vi "New-Main.vi"() -> ()   [LabVIEW 2019]
uses:
  <vilib>/userdefined/High Color/IMAQdx.ctl
  <vilib>/Platform/TimedLoop/XDataNode/nitl_modes.ctl
  <vilib>/Platform/TimedLoop/XDataNode/timing_clust.ctl
  <vilib>/Platform/TimedLoop/XDataNode/wakeup.ctl
  <vilib>/UPVI/lvhdf5/dataset.llb/LVH5D Operation.ctl
  <vilib>/Utility/miscctls.llb/LVRectTypeDef.ctl
  <vilib>/UPVI/lvhdf5/attribute.llb/LVH5A Operation.ctl
  <vilib>/UPVI/lvhdf5/group.llb/H5G_obj_t.ctl
  <vilib>/MakerHub/LINX/Public/Peripherals/Digital/Digital Read 1 Chan.vi
  03419f7f-1d90-4d41-b19f-f0295c63df66.vi
  <vilib>/MakerHub/LINX/Public/Peripherals/PWM/PWM Set Duty Cycle 1 Chan.vi
  <vilib>/UPVI/lvhdf5/identifier.llb/Not an HDF5 Refnum Constant.vi
  <vilib>/MakerHub/LINX/Public/Peripherals/Digital/Digital Read N Chans.vi
  <vilib>/UPVI/lvhdf5/common.llb/To HDF5 Ref.vi
  <vilib>/MakerHub/LINX/Private/Local IO/LinxDigitalRead.vi
  <vilib>/MakerHub/LINX/Public/Utilities/Check Channel.vi
  <vilib>/MakerHub/LINX/Public/Utilities/Open Serial.vi
  <vilib>/MakerHub/LINX/Private/Utilties/Generate Error.vi
  <vilib>/Utility/file.llb/Read Delimited Spreadsheet (DBL).vi
  <vilib>/MakerHub/LINX/Public/Peripherals/PWM/PWM Set Duty Cycle N Chans.vi
  <vilib>/UPVI/lvhdf5/group.llb/OpenCreateGroup (String).vi
  <vilib>/Utility/VariantDataType/GetClusterInfo.vi
  <vilib>/Utility/VariantDataType/GetTypeInfo.vi
  <vilib>/UPVI/lvhdf5/utility.llb/Select HDF5 Dialog.vi
  <vilib>/UPVI/lvhdf5/utility.llb/Select HDF5 Dialog (Object Only).vi
  <vilib>/UPVI/lvhdf5/dataset.llb/Simple H5Dwrite (Variant).vi
  <vilib>/UPVI/lvhdf5/attribute.llb/Write Multiple Attributes.vi
  <vilib>/UPVI/lvhdf5/dataset.llb/H5Dclose.vi
  <vilib>/platform/TimedLoop/XDataNode/XDataNode.xnode
  <vilib>/UPVI/lvhdf5/dataset.llb/Write Dataset with Attributes.xnode
  <vilib>/UPVI/lvhdf5/library.llb/HDF5 Ref.ctl
  <vilib>/UPVI/lvhdf5/attribute.llb/Cluster to Attribute Array.xnode
  <vilib>/UPVI/lvhdf5/dataset.llb/Simple H5Dwrite.xnode
  <vilib>/Platform/TimedLoop/XDataNode/XDNodeRunTimeDep.lvlib
  <vilib>/vision/driver/NI_Vision_Acquisition_Software.lvlib
  <vilib>/MakerHub/LINX/LMH-LINX.lvlib
  <vilib>/Utility/error.llb/Error Cluster From Error Code.vi
  <vilib>/UPVI/lvhdf5/dataset.llb/OpenCreateReplace Dataset by Element Type.vi
  <vilib>/UPVI/lvhdf5/dataspace.llb/H5Sselect_hyperslab.vi
  <vilib>/UPVI/lvhdf5/dataset.llb/H5Dwrite (Variant).vi
  <vilib>/UPVI/lvhdf5/dataset.llb/H5Dget_space.vi
  <vilib>/UPVI/lvhdf5/attribute.llb/private/LVH5AwriteWDTAttrs.vi
  <vilib>/UPVI/lvhdf5/dataspace.llb/H5Sclose.vi
  <vilib>/UPVI/lvhdf5/file.llb/LVH5F Operation.ctl
  <vilib>/UPVI/lvhdf5/utility.llb/Select HDF5 Dialog (File and Object).vi
  <vilib>/Utility/VariantDataType/VariantType.lvlib
panel:
  out "output":dbl[](array[numeric])
  out "motor fb":dbl
  in  "stop":bool
  in  "attributes cluster":T1
  out "CW/CCW":bool
  out "x-y":u32
  out "Trial #":i32[](array[numeric])
  out "stimulus":bool
  out "Timers":dbl[](array[numeric])
  out "% In Exit":dbl[](array[numeric])
  in  "Controls":T2={"Start"=FALSE, "Stop"=FALSE, "success"=FALSE, "set"=FALSE, "fail"=FALSE, "Save Data"=FALSE, "poop count"=0, "Rodent ID"=1, "Correct color"=enum."UV"}
  in  "Settings":T3(tab)
  in  "trial settings":T4={"Num Trials"=6, "Trial Duration (s)"=90, "ITI (s)"=20, "incorrect ITI (s)"=5, "Total Timeout (s)"=900} {"incorrect ITI (s)" min=1 step=1; "Total Timeout (s)" min=1 step=1; "ITI (s)" min=1 step=1; "Num Trials" min=2 step=2; "Trial Duration (s)" min=1 step=1}
  in  "dir":T5={"Data Output Directory"=path "D:/pdroft", "Session Name"="default"}
  in  "habituation":bool
  in  "feedback":T6={"motor feedback mode"=enum."constant", "min motor feedback"=0.1, "max motor feedback"=0.5, "max led feedback"=1.0, "colormap"=path "C:/Program Files/PDROFT/data/colormap_test121219e.txt"} {"min motor feedback" min=0.0 max=1.0; "max led feedback" min=0.0 max=1.0; "max motor feedback" min=0.0 max=1.0}
  in  "ROI":T7
  in  "vid bandpass":T8={"low1"=1, "high1"=7, "low2"=27, "high2"=100}
  in  "I/O":T10={"Vid In"="cam0", "record raw video?"=FALSE, "record filtered video?"=FALSE, "microcontroller Serial Port"="COM4", "Disable physical start butn"=FALSE}
  in  "exits":T11={"hab scale"=0.7, "exit radius (cm)"=12.5, "% required in exit"=42.0}
  in  "save settings to ini at close":bool
  in  "load settings from ini at start":bool
  out "Image":T12(plugin-control)
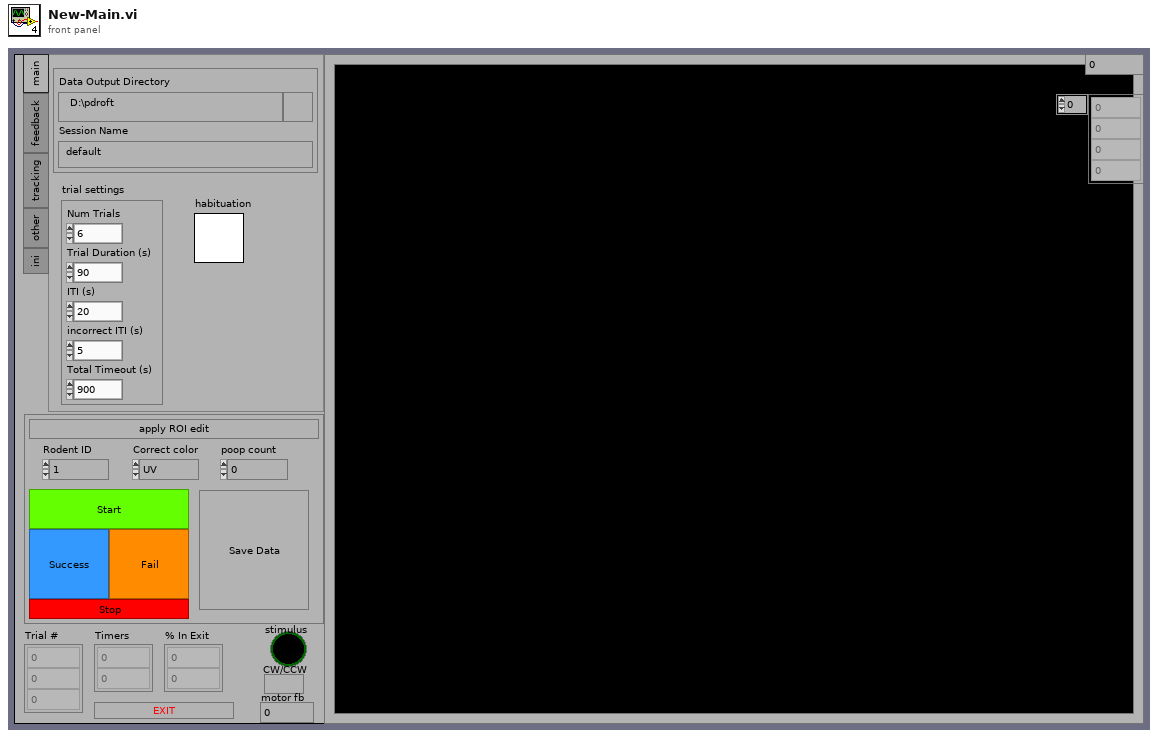
[diagram p1: front panel]
types:
  T1 = cluster{"timestamp":string, "ID":string, "correct color":string, "poop count":string, "trial settings":string, "motor settings":string, "max led fb":string, "colormap":string, "vid bandpass":string, "exit settings":string, "platform":string, "px2cm":string}
  T2 = cluster{"Start":bool, "Stop":bool, "success":bool, "set":bool, "fail":bool, "Save Data":bool, "poop count":i8, "Rodent ID":i32, "Correct color":enum16{"UV", "Green"}}
  T3 = enum32{"main", "feedback", "tracking", "other", "ini"}
  T4 = cluster{"Num Trials":i32, "Trial Duration (s)":i32, "ITI (s)":i32, "incorrect ITI (s)":i32, "Total Timeout (s)":i32}
  T5 = cluster{"Data Output Directory":path, "Session Name":string}
  T6 = cluster{"motor feedback mode":enum16{"constant", "time still"}, "min motor feedback":dbl, "max motor feedback":dbl, "max led feedback":dbl, "colormap":path}
  T7 = cluster{"Global Rectangle":i32[], "Contours":cluster{"Contour Type":u32, "ROI Type":u32, "Points":i32[]}[]}
  T8 = cluster{"low1":i32, "high1":i32, "low2":i32, "high2":i32}
  T9 = typedef "IMAQdx.ctl" = refnum<k21>
  T10 = cluster{"Vid In":T9, "record raw video?":bool, "record filtered video?":bool, "microcontroller Serial Port":refnum<visa-resource-name>, "Disable physical start butn":bool}
  T11 = cluster{"hab scale":dbl, "exit radius (cm)":dbl, "% required in exit":dbl}
  T12 = typedef "IMAQ Image.ctl" = refnum<image>
  T13 = typedef "XDNodeRunTimeDep.lvlib/nitl_modes.ctl" = enum32{"No Change", "Process missed periods, maintain original phase", "Discard missed periods, maintain original phase", "Process missed periods, ignore original phase", "Discard missed periods, ignore original phase"}
  T14 = enum8{"Enabled", "Disabled", "Disabled and Grayed Out"}
  T15 = typedef "LVRectTypeDef.ctl" = cluster{"Left":i16, "Top":i16, "Right":i16, "Bottom":i16}
  T16 = cluster{"Behavior":enum32{"Invalid", "Default", "Floating", "Floating/Auto-Hide", "Modal"}, "Position":T15, "Center":bool, "Title":string}
  T17 = typedef "LVH5F Operation.ctl" = enum16{"open", "open or create", "create or replace", "create or replace (with confirmation)", "create", "open (read only)"}
  T18 = typedef "LVH5D Operation.ctl" = enum16{"open", "replace", "create", "open or create", "create or replace", "create or replace with confirmation"}
  T19 = typedef "H5G_obj_t.ctl" = i32
  T20 = cluster{"Object Types (any)":T19[], "Object Pattern":string}
  T21 = typedef "LVH5A Operation.ctl" = enum16{"open", "replace", "create", "open or create", "create or replace", "create or replace with confirmation"}
  T22 = cluster{"Session Timer":dbl, "Trial Timer":dbl, "Trial #":dbl, "Correction #":dbl, "Omission":dbl, "CentroidX":dbl, "CentroidY":dbl, "%Correct":dbl, "%Incorrect":dbl, "R":dbl, "G":dbl, "B":dbl, "W":dbl, "M":dbl, "Total":dbl}
  T23 = typedef "XDNodeRunTimeDep.lvlib/timing_clust.ctl" = cluster{"Expected End [f-1]":u64, "Actual End [f-1]":u64, "Finished Late? [f-1]":bool, "Expected End [i-1]":u64, "Actual End [i-1]":u64, "Finished Late? [i-1]":bool, "Expected Start [i]":u64, "Actual Start [i]":u64, "Expected Start [f]":u64, "Actual Start [f]":u64, "Source Name":string, "Structure Name":string, "Period":i64, "Deadline":i64, "Offset":i64, "Start":i64, "Priority":i32, "Timeout":i32, "Mode":T13, "Wakeup Reason":T24, "Error":errorcluster, "Source Type":string, "Secondary Source Type":string, "Global End Time":u64, "Global Start Time":u64, "Frame Duration":u64, "Iteration Duration":u64, "Assigned CPU":i32, "I/O Scan Engine Mode":u32}
  T24 = typedef "XDNodeRunTimeDep.lvlib/wakeup.ctl" = enum32{"Normal", "Aborted", "Asynchronous wakeup", "Timing source error", "Timed loop error", "Timeout"}
  T25 = enum32{"invalid app kind", "Development System", "Run Time System", "Student Edition", "Embedded LabVIEW", "Evaluation", "Custom"}
  T26 = typedef "Image Type" = u32
  T27 = typedef "LMH-LINX.lvlib/LINX Ref.ctl" = cluster{"IO":T28, "Interface":T29, "LINX Device Config":T30}
  T28 = typedef "LMH-LINX.lvlib/Platform.ctl" = enum16{"Remote", "Local"}
  T29 = typedef "LMH-LINX.lvlib/Interface.ctl" = enum16{"Serial", "TCP"}
  T30 = typedef "LMH-LINX.lvlib/Device.lvlib/LINX Device Config.ctl" = cluster{"Interface":T29, "COM Port":refnum<visa-resource-name>, "TCP Configuration":T31, "Device Family":u8, "Device ID":u8, "Device Name":string, "TCP Ref":refnum<k5>, "Channels":T32}
  T31 = typedef "LMH-LINX.lvlib/Device.lvlib/TCP Config.ctl" = cluster{"IP Address":string, "Port":u16}
  T32 = typedef "LMH-LINX.lvlib/Channels.ctl" = cluster{"DI":u8[], "DO":u8[], "AI":u8[], "AO":u8[], "PWM":u8[], "QE":u8[], "UART":u8[], "I2C 2":u8[], "SPI":u8[], "CAN":u8[], "Servo":u8[], "AI Ref (V)":dbl, "AI Resolution (Bits)":u8, "AO Ref (V)":dbl, "AO Resolution (Bits)":u8}
  T33 = cluster{"Trial#":dbl, "Correction#":dbl, "Omission":dbl, "CorrectX":dbl, "CorrectY":dbl, "IncorrectX":dbl, "IncorrectY":dbl, "CW/CCW":dbl}
  T34 = typedef "IMAQ AVI2 Refnum.ctl" = refnum<k20>
  T35 = cluster{"Trial#":dbl, "Correction#":dbl, "Omission":dbl, "CorrectX":dbl, "CorrectY":dbl, "IncorrectX":dbl, "IncorrectY":dbl, "CW/CCW":dbl}[]
  T36 = cluster{"center":dbl[], "center":dbl[], "hab rad":dbl, "Timers":dbl[]}
  T37 = cluster{"px2cm":dbl, "center":dbl[], "rad":dbl, "hab rad":dbl, "exit rad":dbl}
  T38 = cluster{"correct exit":dbl[], "incorrect exit":dbl[], "exit rad":dbl, "exit angles":dbl[]}
  T39 = typedef "HDF5 Ref.ctl" = refnum<k1>
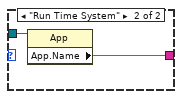
[diagram p3: hidden frame]
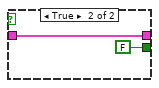
[diagram p4: hidden frame]
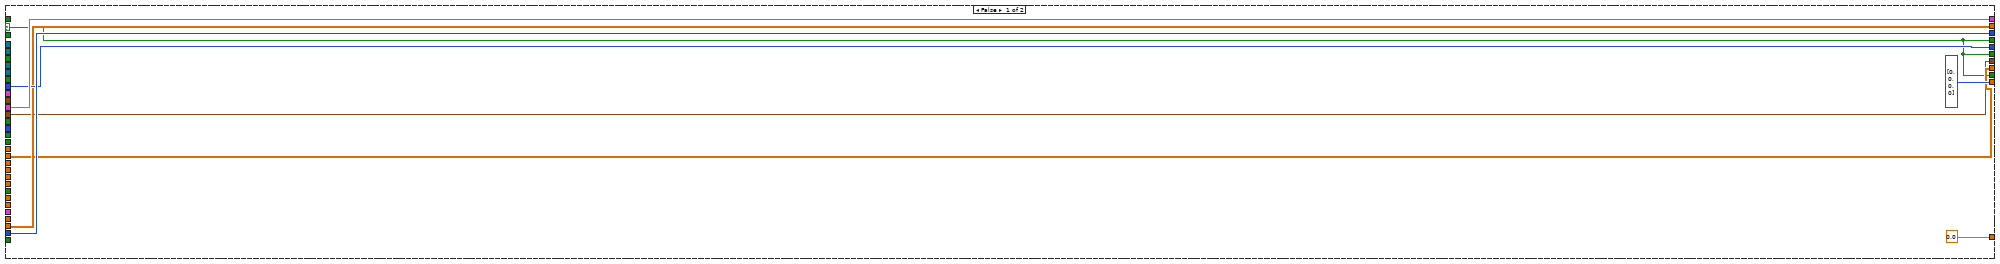
[diagram p9: hidden frame]
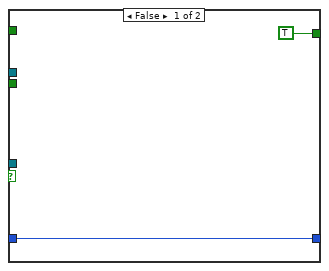
[diagram p11: hidden frame]
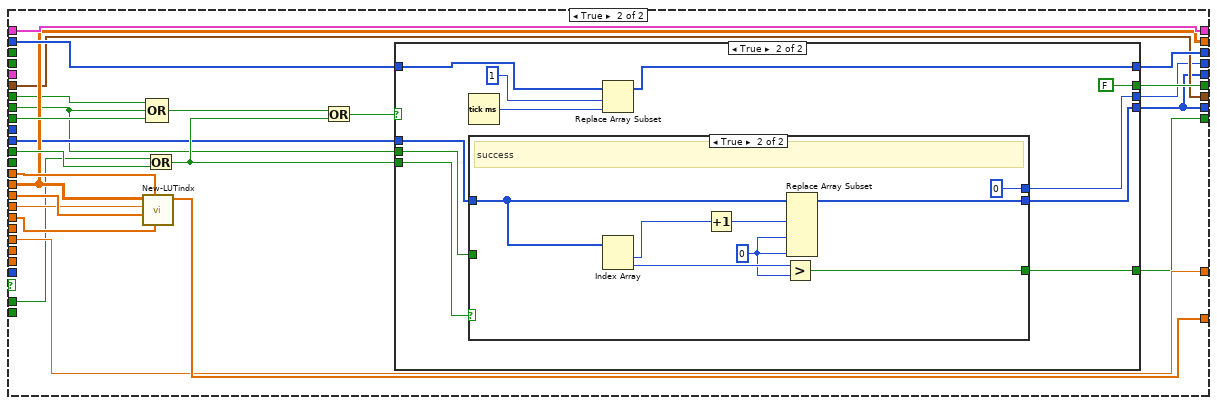
[diagram p16: hidden frame]
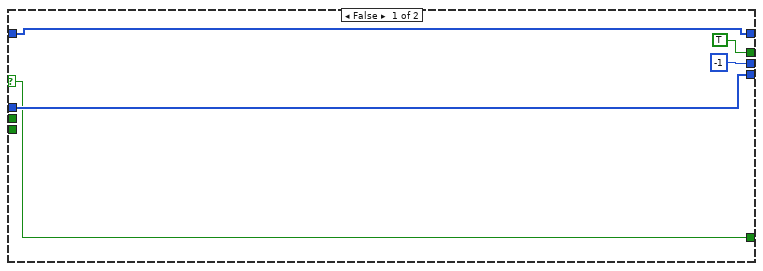
[diagram p17: hidden frame]
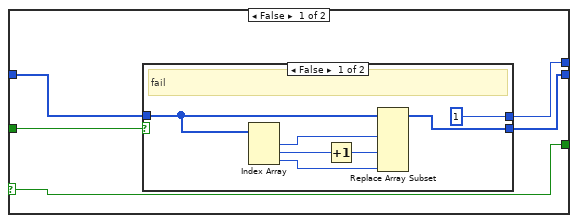
[diagram p18: hidden frame]
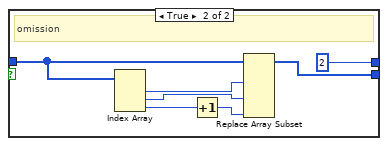
[diagram p19: hidden frame]
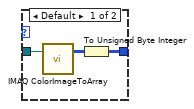
[diagram p20: hidden frame]
diagram:
  n1 = flat-sequence {
    tunnel: [w5] -> w2
    tunnel: [w4] -> w1
    tunnel: w2 -> [w1170]
    tunnel: w1 -> [w1169]
    frame #0 {
      n2 = property class="App"() -> (reference out=w8:refnum<vi>, "App.Kind"=w9:T25)  [unwired: 2 in, 1 out]
      n3 = case shown="\"Development System\", Default" w9 {
        tunnel: w8 -> [_ w16]
        tunnel: [w14 w15] -> w6
        frame "Development System", Default {
          n4 = property class="VI"() -> ("Name"=w14:string)  [unwired: 2 in, 2 out]
        }
        frame "Run Time System" {
          n5 = property class="App"(reference=w16) -> ("App.Name"=w15:string)  [unwired: 1 in, 2 out]
        }
      }
      n6 = control-ref of="Settings"() -> (w7:refnum<vi>)
      n7 = property class="TabCtl (strict)"(reference=w7) -> ("Pages"=w4:refnum<vi>[])  [unwired: 1 in, 2 out]
      n8 = call "Generate INI file path.vi"("VI or App Name"=w6) -> ("appended path"=w5:path)
      n9 = case shown="True" "load settings from ini at start" {
        tunnel: w5 -> [_ w11]
        tunnel: w4 -> [_ w10]
        frame False {
        }
        frame True {
          n10 = for {
            tunnel: w11 -> [w13]
            tunnel: w10 -> [w12] mode=indexing
            n11 = call "my Read Controls on Tab from Config File.vi"("Page Refnum"=w12, "configuration file path"=w13) -> ()  [unwired: 4 in, 2 out]
          }
        }
      }
    }
    frame #1 {
      n12 = control-ref of="Image"() -> (w18:refnum<vi>)
      n13 = property class="ImageControl"(reference=w18, "ROI"="ROI") -> ()  [unwired: 1 in, 2 out]
    }
    frame #2 {
      w33 = dbl[] [0.0, 0.0] ("Timers")
      w27 = FALSE
      w36 = T26 0 items=["Grayscale (U8)", "Grayscale (I16)", "Grayscale (SGL)", "Complex (CSG)", "RGB (U32)", "HSL (U32)", "RGB (U64)", "Grayscale (U16)"] ("Image Type")
      n14 = property on="Timers" class="Arr (strict)"("Value"=w33) -> ()  [unwired: 2 in, 2 out]
      n15 = property on="% In Exit" class="Arr (strict)"("Value"=w33) -> ()  [unwired: 2 in, 2 out]
      n16 = Unbundle("I/O") -> ("Vid In"=w47:T9, "record raw video?"=w38:bool, "record filtered video?"=w22:bool, "microcontroller Serial Port"=w23:refnum<visa-resource-name>, "Disable physical start butn"=w19:bool)
      n17 = call-poly <vilib>:"Open.vi"("Serial Port"=w23) -> ("Error Out"=w26:errorcluster, "LINX Resource"=w29:T27)  [unwired: 8 in, 1 out]
      n18 = call <vilib>:"IMAQdx Open Camera.vi"("Session In"=w47) -> ("Session Out"=w48:T9)  [unwired: 9 in, 1 out]
      n19 = call <vilib>:"IMAQdx Configure Grab.vi"("Session In"=w48) -> ("Session Out"=w43:T9)  [unwired: 9 in, 1 out]
      n20 = call <vilib>:"General Error Handler.vi"("[error source] (\" \")"="microcontroller connection" ("[error source] (\" \")"), "error in (no error)"=w26) -> ("error?"=w25:bool)  [unwired: 9 in, 4 out]
      n21 = call "IMAQ Create"("Image Name"="untitled0", "Image Type"=w36) -> ("New Image"=w42:T12)  [unwired: 3 in, 1 out]
      n22 = call "IMAQ Create"("Image Name"="untitled1", "Image Type"=w36) -> ("New Image"=w35:T12)  [unwired: 3 in, 1 out]
      n23 = CPU Information() -> (4:w30:i32)  [unwired: 3 out]
      n24 = node-c288(i64 100 ("Period"), nitl_modes."Process missed periods, maintain original phase" ("Mode")) -> (w50:T23)
      n25 = timed-loop {
        timing: w50 -> [_]
        timing-out: [_] -> w49
        tunnel: "Settings" -> [_]
        tunnel: w43 -> [w155]
        tunnel: w42 -> [w153]
        shift-right: [w114] -> _
        shift-left: w27 -> [w131]
        tunnel: [w152] -> w40
        tunnel: [w154] -> w41
        shift-right: [w113] -> _
        shift-left: w27 -> [w151]
        tunnel: w38 -> [w140]
        shift-right: [w145] -> _
        shift-left: _ -> [w146]
        shift-right: [w143] -> _
        shift-left: _ -> [w144]
        shift-right: [w89] -> _
        shift-left: _ -> [w81]
        tunnel: w35 -> [w150]
        tunnel: [w63] -> w34
        shift-right: [w148] -> _
        shift-left: _ -> [w149]
        shift-right: [w100] -> _
        shift-left: _ -> [w101]
        shift-right: [w112] -> _
        shift-left: i32[] [0, 0, 0] -> [w132]
        shift-right: [w111] -> _
        shift-left: i32[] [0, 0] -> [w147]
        tunnel: w30 -> [w137]
        tunnel: w29 -> [w69]
        tunnel: [w108] -> w28
        tunnel: w25 -> [w70]
        shift-right: [w90] -> _
        shift-left: _ -> [w99]
        shift-right: [w86] -> _
        shift-left: _ -> [w88]
        tunnel: w22 -> [w65]
        shift-right: [w64] -> _
        shift-left: _ -> [w66]
        shift-right: [w59] -> _
        shift-left: i32[] [0, 0, 1, 1] -> [w60]
        tunnel: w19 -> [w52]
        stop <- "stop" stop-if-true
        n26 = node-c288() -> ()  [unwired: 1 in, 1 out]
        n27 = Or(x=w52, y=w70) -> (x .or. y?=w53:bool)
        n28 = Unbundle("Controls") -> ("Start"=w135:bool, "Stop"=w115:bool, "success"=w119:bool, "set"=w116:bool, "fail"=w118:bool, "Save Data"=w134:bool, "Rodent ID"=w138:i32, "Correct color"=w105:enum16{"UV", "Green"})  [unwired: 1 out]
        n29 = case shown="False" w53 {
          tunnel: w69 -> [w159 w161]
          tunnel: [w158 w161] -> w58
          tunnel: [w157 FALSE ("DI Value")] -> w68
          frame False {
            n30 = call-poly <vilib>:"Digital Read.vi"("DI Channel"=u8 4, "LINX Resource"=w159) -> ("DI Value"=w157:bool, "LINX Resource"=w158:T27)  [unwired: 7 in, 1 out]
          }
          frame True {
          }
        }
        n31 = Or(x=w68, y=w135) -> (x .or. y?=w71:bool)
        n32 = Equal?(x=enum16{"UV", "Green"}."Green" ("Correct color"), y=w105) -> (x = y?=w102:bool)
        n33 = Compound Arithmetic op=AND(w134, invert w131) -> (w133:bool)
        n34 = property on="Start" class="Bool"() -> ("DisabledEnum"=w57:T14)  [unwired: 2 in, 2 out]
        n35 = Not Equal?(x=w57, y=T14."Disabled and Grayed Out" ("Disabled")) -> (x != y?=w55:bool)
        n36 = Compound Arithmetic op=AND(w71, invert w131, w55) -> (w54:bool)
        n37 = First Call?() -> (First Call?: T/F=w139:bool)
        n38 = feedback #1() -> (w96:string)  [unwired: 1 in]
        n39 = case "start" shown="True" w54 {
          selector: w54 -> [_ w494]
          tunnel: [w456 w494] -> w136
          tunnel: w140 -> [_ w498]
          tunnel: "dir" -> [_ w499]
          tunnel: [w458 w489] -> w145
          tunnel: w146 -> [w458 w488]
          tunnel: w147 -> [w457 w493]
          tunnel: [w457 w492] -> w110
          tunnel: [w455 i32[] [1, 0, 0]] -> w109
          tunnel: w138 -> [_ w475]
          tunnel: w131 -> [w456 _]
          tunnel: w132 -> [w455 _]
          tunnel: w99 -> [w454 w481]
          tunnel: [w454 w484] -> w98
          tunnel: [w453 w486] -> w97
          tunnel: w96 -> [w453 _]
          tunnel: w88 -> [w452 w483]
          tunnel: [w452 w482] -> w87
          tunnel: w65 -> [_ w474]
          tunnel: [w451 w473] -> w64
          tunnel: w66 -> [w451 w472]
          tunnel: "trial settings" -> [_ w471]
          tunnel: [w450 w462] -> w59
          tunnel: w60 -> [w450 _]
          frame False {
          }
          frame True {
            w461 = 0.0
            n40 = Unbundle By Name(w471) -> ("Num Trials"=w470:i32)
            n41 = Array Size(array=w481) -> (size(s)=w480:i32[])
            n42 = Index Array(array=w483) -> (element=w459:T33)  [unwired: 1 in]
            n43 = Unbundle(w499) -> ("Data Output Directory"=w477:path, "Session Name"=w476:string)
            n44 = Tick Count (ms)() -> (millisecond timer value=w491:u32)
            n45 = property on="Start" class="Bool"("DisabledEnum"=T14."Disabled and Grayed Out" ("Disabled")) -> ()  [unwired: 2 in, 2 out]
            n46 = case shown="True" w474 {
              tunnel: w475 -> [_ w509]
              tunnel: w477 -> [_ w508]
              tunnel: w476 -> [_ w507]
              tunnel: [w500 w503] -> w473
              tunnel: w472 -> [w500 _]
              frame False {
              }
              frame True {
                n47 = Concatenate Strings(w507, "_filt" ("string")) -> (w502:string)
                n48 = call "check vid path.vi"("Trial #"=w509, "Experiment Name"=w502, "Data Output Directory"=w508) -> ("appended path"=w506:path)  [unwired: 8 in]
                n49 = call "IMAQ AVI2 Create"("Codec"="Motion JPEG (NI Vision)", "Frames Per Second"=u32 10, "AVI Path"=w506) -> ("AVI Refnum"=w503:T34)  [unwired: 7 in, 1 out]
              }
            }
            n50 = case shown="True" w498 {
              tunnel: w475 -> [_ w517]
              tunnel: w477 -> [_ w516]
              tunnel: w476 -> [_ w515]
              tunnel: [w510 w511] -> w489
              tunnel: w488 -> [w510 _]
              frame False {
              }
              frame True {
                n51 = call "check vid path.vi"("Trial #"=w517, "Experiment Name"=w515, "Data Output Directory"=w516) -> ("appended path"=w514:path)  [unwired: 8 in]
                n52 = call "IMAQ AVI2 Create"("Codec"="Motion JPEG (NI Vision)", "Frames Per Second"=u32 10, "AVI Path"=w514) -> ("AVI Refnum"=w511:T34)  [unwired: 7 in, 1 out]
              }
            }
            n53 = Replace Array Subset(array=w493, new element #1=w491, new element #2=w491) -> (w492:i32[])  [unwired: 2 in]
            n54 = Index Array(array=w480) -> (element #2=w479:i32)  [unwired: 2 in, 1 out]
            n55 = Bundle(cluster=w459, "Trial#"=w461, "Correction#"=w461, "Omission"=w461, "CorrectX"=w461, "CorrectY"=w461, "IncorrectX"=w461, "IncorrectY"=w461, "CW/CCW"=w461) -> (w460:T33)
            n56 = Divide(x=w470, y=2) -> (x/y=w468:dbl)
            n57 = Build Array(w460) -> (w482:T35)
            n58 = Initialize Array(0, w468) -> (w465:i32[])
            n59 = Initialize Array(1, w468) -> (w464:i32[])
            n60 = Get Date/Time String(want seconds? (F)=w494) -> (date string=w497:string, time string=w496:string)  [unwired: 2 in]
            n61 = Build Array (concatenate)(w465, w464) -> (w463:i32[])
            n62 = Format Into String(format string="%s %s", w497, w496) -> (resulting string=w486:string)  [unwired: 2 in, 1 out]
            n63 = call "Shuffle 1D Array.vim"("array"=w463) -> ("shuffled array"=w462:i32[])  [unwired: 4 in]
            n64 = Initialize Array(0.0 ("element"), 1 ("dimension size"), w479) -> (w484:dbl[][])
          }
        }
        n65 = feedback-in #1(w97) -> ()
        n66 = Or(x=w139, y=w116) -> (x .or. y?=w117:bool)
        n67 = call <vilib>:"IMAQdx Grab2.vi"("Wait for Next Buffer? (Yes)"=FALSE, "Image In"=w153, "Session In"=w155) -> ("Image Out"=w152:T12, "Session Out"=w154:T9)  [unwired: 5 in, 2 out]
        n68 = call "IMAQ GetImageInfo"("Image"=w152) -> ("Y Resolution"=w141:i32, "X Resolution"=w142:i32, "Image Type"=w130:T26)  [unwired: 3 in, 5 out]
        n69 = case shown="0..2" w130 {
          tunnel: w152 -> [w446 w449]
          tunnel: [w445 w448] -> w129
          frame Default {
            n70 = call "IMAQ ColorImageToArray"("Image"=w446) -> ("Image Pixels (U32)"=w447:u32[][])  [unwired: 3 in, 2 out]
            n71 = To Unsigned Byte Integer(number=w447) -> (unsigned 8bit integer=w445:u8[][])
          }
          frame 0..2 {
            n72 = call "IMAQ ImageToArray"("Image"=w449) -> ("Image Pixels (U8)"=w448:u8[][])  [unwired: 3 in, 4 out]
          }
        }
        n73 = Unbundle(w149) -> ("correct exit"=w122:dbl[], "incorrect exit"=w124:dbl[], "exit rad"=w123:dbl, "exit angles"=w120:dbl[])
        n74 = call "New2-Track.vi"("vid bandpass"="vid bandpass", "mask"=w144, "# of logical processors"=w137, "correct"=w124, "incorrect"=w122, "exit rad"=w123, "X Resolution"=w142, "Y Resolution"=w141, "Image Pixels (U8)"=w129) -> ("%inexit"=w127:dbl[], "centroid"=w93:dbl[], "Numeric"=w62:i32, "vid"=w128:u8[][])  [unwired: 3 in]
        "% In Exit" <- w127
        n75 = feedback-in #2(w93) -> ()
        n76 = feedback #2() -> (w92:dbl[])  [unwired: 1 in]
        n77 = call "dist btwn 2 points.vi"("coord pair 2"=w92, "coord pair1"=w93) -> ("dist"=w91:dbl)  [unwired: 9 in]
        n78 = Unbundle(w81) -> ("center"=w80:dbl[], "rad"=w78:dbl, "hab rad"=w79:dbl, "exit rad"=w77:dbl)  [unwired: 1 out]
        n79 = call "New-VidOverlays.vi"("exit rad"=w123, "center"=w80, "correct"=w124, "hab rad"=w79, "incorrect"=w122, "vid"=w128, "centroid"=w93, "Refnum in"=w150) -> ("Refnum out"=w63:T12)  [unwired: 3 in]
        "Image" <- w63
        n80 = Unbundle By Name("exits") -> ("% required in exit"=w126:dbl)
        n81 = Bundle("center"=w80, "center"=w80, "hab rad"=w79, "Timers"=dbl[] [0.0, 0.0]) -> (w125:T36)  [unwired: 1 in]
        n82 = feedback #3() -> (w104:dbl[][])  [unwired: 1 in]
        n83 = case "edit ROI" shown="True" w117 {
          tunnel: [w519 w532] -> w143
          tunnel: "exits" -> [_ w531]
          tunnel: [w520 w530] -> w89
          tunnel: w81 -> [w520 _]
          tunnel: w144 -> [w519 _]
          tunnel: [w518 w522] -> w103
          tunnel: w104 -> [w518 _]
          tunnel: "feedback" -> [_ w526]
          tunnel: w142 -> [_ w524]
          tunnel: w141 -> [_ w523]
          frame False {
          }
          frame True {
            n84 = Unbundle By Name(w526) -> ("colormap"=w525:path, "max led feedback"=w521:dbl)
            n85 = call-poly <vilib>:"Read Delimited Spreadsheet.vi"("file path (dialog if empty)"=w525) -> ("all rows"=w529:dbl[][], "error out"=w528:errorcluster)  [unwired: 9 in, 4 out]
            n86 = property on="Image" class="ImageControl"() -> ("ROI"=w535:T7)  [unwired: 2 in, 2 out]
            n87 = call <vilib>:"Simple Error Handler.vi"("error source (\" \")"="error loading colormap" ("error source (\" \")"), "error in (no error)"=w528) -> ()  [unwired: 3 in, 5 out]
            n88 = property on="ROI" class="Clust (strict)"("Value"=w535) -> ()  [unwired: 2 in, 2 out]
            n89 = Multiply(x=w529, y=w521) -> (x*y=w522:dbl[][])
            n90 = call "New-ROIstuff.vi"("exits position"=w531, "X Resolution"=w524, "rad scale"=1.1 ("radius"), "Y Resolution"=w523, "plat diam(cm)"=121.92, "ROI"=w535) -> ("platform"=w530:T37, "Array"=w532:bool[][])  [unwired: 4 in]
          }
        }
        n91 = feedback-in #3(w103) -> ()
        n92 = case "Session Running" shown="True" w136 {
          selector: w136 -> [w187 _]
          tunnel: w140 -> [_ w274]
          tunnel: w152 -> [_ w290]
          tunnel: w151 -> [_ w201]
          tunnel: w145 -> [_ w273]
          tunnel: w127 -> [_ w224]
          tunnel: w126 -> [_ w225]
          tunnel: w93 -> [_ w259]
          tunnel: w80 -> [_ w289]
          tunnel: w79 -> [_ w266]
          tunnel: w77 -> [_ w288]
          tunnel: w125 -> [w195 w286]
          tunnel: [w195 w287] -> w148
          tunnel: w149 -> [_ w285]
          tunnel: "trial settings" -> [_ w217]
          tunnel: w120 -> [_ w284]
          tunnel: w78 -> [_ w283]
          tunnel: w110 -> [w194 w268]
          tunnel: w109 -> [w193 w258]
          tunnel: w119 -> [_ w278]
          tunnel: w118 -> [_ w277]
          tunnel: w115 -> [_ w276]
          tunnel: [w187 w272] -> w114
          tunnel: [w187 w271] -> w113
          tunnel: [w193 w270] -> w112
          tunnel: [w194 w269] -> w111
          tunnel: [u8[] [0, 0, 0, 0] ("output") w255] -> w73
          tunnel: [0.0 w254] -> w107
          tunnel: "feedback" -> [_ w265]
          tunnel: w101 -> [_ w264]
          tunnel: w103 -> [w190 w263]
          tunnel: w102 -> [_ w262]
          tunnel: [w190 w261] -> w100
          tunnel: w98 -> [w189 w257]
          tunnel: w91 -> [_ w248]
          tunnel: [w189 w242] -> w90
          tunnel: [w188 w236] -> w86
          tunnel: w87 -> [w188 w235]
          tunnel: "habituation" -> [_ w216]
          tunnel: w65 -> [_ w207]
          tunnel: w64 -> [_ w206]
          tunnel: w63 -> [_ w205]
          tunnel: w62 -> [_ w204]
          tunnel: w59 -> [_ w203]
          tunnel: w58 -> [_ _]
          tunnel: w54 -> [_ _]
          tunnel: [w187 w198] -> w51
          frame False {
          }
          frame True {
            w215 = 300
            w212 = 1000
            n93 = case shown="True" w274 {
              tunnel: w273 -> [_ w305]
              tunnel: w290 -> [_ w304]
              frame False {
              }
              frame True {
                n94 = call "IMAQ AVI2 Write Frame"("Image"=w304, "AVI Refnum"=w305) -> ()  [unwired: 7 in, 3 out]
              }
            }
            n95 = case shown="True" w207 {
              tunnel: w206 -> [_ w292]
              tunnel: w205 -> [_ w291]
              frame False {
              }
              frame True {
                n96 = call "IMAQ AVI2 Write Frame"("Image"=w291, "AVI Refnum"=w292) -> ()  [unwired: 7 in, 3 out]
              }
            }
            n97 = Unbundle By Name(w265) -> ("min motor feedback"=w243:dbl, "max motor feedback"=w249:dbl, "motor feedback mode"=w252:enum16{"constant", "time still"})
            n98 = Index Array(array=w258) -> (element=w280:i32)  [unwired: 1 in]
            n99 = Greater?(x=w224, y=w225) -> (0:w223:bool[])
            n100 = Less?(x=w248, y=5.0) -> (x < y?=w241:bool)
            n101 = Bundle(cluster=w217, "Num Trials"=1, "Trial Duration (s)"=w215, "ITI (s)"=w215, "incorrect ITI (s)"=w215, "Total Timeout (s)"=w215) -> (w219:T4)
            n102 = Select(t=w219, s=w216, f=w217) -> (s? t:f=w218:T4)
            n103 = feedback #4(w243) -> (w245:dbl)
            n104 = Index Array(array=w223) -> (element #1=w222:bool, element #2=w221:bool)  [unwired: 2 in]
            n105 = Select(t=0.01, s=w241, f=-0.02) -> (s? t:f=w240:dbl)
            n106 = Add(x=w240, y=w245) -> (x+y=w246:dbl)
            n107 = Equal?(x=enum16{"constant", "time still"}."time still" ("motor feedback mode"), y=w252) -> (x = y?=w251:bool)
            n108 = Index Array(array=w268) -> (element #1=w230:i32, element #2=w229:i32)  [unwired: 2 in]
            n109 = Unbundle(w218) -> ("Num Trials"=w228:i32, "Trial Duration (s)"=w227:i32, "ITI (s)"=w226:i32, "incorrect ITI (s)"=w213:i32, "Total Timeout (s)"=w214:i32)
            n110 = Tick Count (ms)() -> (millisecond timer value=w267:u32)
            n111 = Greater?(x=w280, y=w228) -> (0:w279:bool)
            n112 = Multiply(x=w214, y=w212) -> (x*y=w233:i32)
            n113 = Multiply(x=w213, y=w212) -> (x*y=w211:i32)
            n114 = Multiply(x=w226, y=w212) -> (x*y=w231:i32)
            n115 = Multiply(x=w227, y=w212) -> (x*y=w232:i32)
            n116 = Subtract(x=w267, y=w230) -> (x-y=w210:u32)
            n117 = In Range and Coerce(upper limit=w249, x=w246, lower limit=w243) -> (coerced(x)=w244:dbl)  [unwired: 1 out]
            n118 = feedback-in #4(w244) -> ()
            n119 = Subtract(x=w267, y=w229) -> (x-y=w209:u32)
            n120 = Greater?(x=w210, y=w233) -> (0:w281:bool)
            n121 = Greater?(x=w209, y=w211) -> (0:w208:bool)
            n122 = Greater?(x=w209, y=w231) -> (0:w282:bool)
            n123 = Greater?(x=w209, y=w232) -> (0:w202:bool)
            n124 = Select(t=w244, s=w251, f=w249) -> (s? t:f=w253:dbl)
            n125 = Build Array(w210, w209) -> (w234:u32[])
            n126 = Divide(x=w234, y=w212) -> (x/y=w260:dbl[])
            "Timers" <- w260
            n127 = Compound Arithmetic op=OR(w276, w281, w279) -> (w275:bool)
            n128 = feedback #5(-1) -> (w200:i32)
            n129 = case "Trial Running" shown="False" w201 {
              selector: w201 -> [w310 _]
              tunnel: w259 -> [w352 w399]
              tunnel: w289 -> [w351 w398]
              tunnel: w288 -> [w350 _]
              tunnel: [w349 w401] -> w287
              tunnel: w286 -> [w348 _]
              tunnel: w285 -> [_ w401]
              tunnel: w284 -> [_ w400]
              tunnel: w266 -> [w346 _]
              tunnel: w283 -> [_ w397]
              tunnel: w202 -> [_ w380]
              tunnel: w282 -> [w326 _]
              tunnel: w278 -> [_ w393]
              tunnel: w277 -> [_ w392]
              tunnel: [w347 w391] -> w271
              tunnel: w258 -> [w318 w385]
              tunnel: [w318 w381] -> w270
              tunnel: w268 -> [w345 w390]
              tunnel: [w344 w389] -> w269
              tunnel: [w314 w388] -> w255
              tunnel: w253 -> [w338 w387]
              tunnel: [w336 w387] -> w254
              tunnel: w264 -> [w340 w386]
              tunnel: w263 -> [w343 _]
              tunnel: w262 -> [w342 _]
              tunnel: [w341 w386] -> w261
              tunnel: [w339 w381] -> w256
              tunnel: [w335 w384] -> w236
              tunnel: w235 -> [w334 w384]
              tunnel: w222 -> [w331 w383]
              tunnel: w221 -> [_ w382]
              tunnel: w216 -> [w333 _]
              tunnel: w208 -> [w325 _]
              tunnel: w203 -> [w322 _]
              tunnel: [w312 w379] -> w197
              tunnel: w200 -> [w312 _]
              tunnel: [w310 w378] -> w198
              frame False {
                n130 = Index Array(array=w318) -> (element=w323:i32)  [unwired: 1 in]
                n131 = Not(x=w331) -> (.not. x?=w329:bool)
                n132 = Equal?(x=w312, y=1) -> (x = y?=w308:bool)
                n133 = Equal?(x=w312, y=2) -> (x = y?=w306:bool)
                n134 = Select(t=w329, s=w333, f=w308) -> (s? t:f=w330:bool)
                n135 = Or(x=w306, y=w308) -> (x .or. y?=w307:bool)
                n136 = And(x=w329, y=w333) -> (x .and. y?=w332:bool)
                n137 = Decrement(x=w323) -> (x-1=w321:i32)
                n138 = Select(t=w325, s=w307, f=w326) -> (s? t:f=w309:bool)
                n139 = Index Array(array=w322, index=w321) -> (element=w320:i32)
                n140 = Compound Arithmetic op=OR(w332, w306) -> (w324:bool)
                n141 = Select(t=w338, s=w330, f=0.0) -> (s? t:f=w336:dbl)
                n142 = And(x=w329, y=w309) -> (x .and. y?=w353:bool)
                n143 = Equal To 0?(x=w320) -> (x = 0?=w319:bool)
                n144 = Negate(x=w318) -> (-x=w339:i32[])
                n145 = case "Next Stim" shown="True" w353 {
                  selector: w353 -> [w357 w372]
                  tunnel: w352 -> [_ w376]
                  tunnel: w351 -> [_ w377]
                  tunnel: w346 -> [_ w375]
                  tunnel: w350 -> [_ w374]
                  tunnel: [w358 w373] -> w349
                  tunnel: w348 -> [w358 _]
                  tunnel: [w357 w372] -> w347
                  tunnel: w345 -> [w356 w369]
                  tunnel: [w356 w368] -> w344
                  tunnel: w343 -> [_ w367]
                  tunnel: w342 -> [_ w366]
                  tunnel: [w355 w365] -> w341
                  tunnel: w340 -> [w355 _]
                  tunnel: [w354 w363] -> w335
                  tunnel: w334 -> [w354 w362]
                  tunnel: w319 -> [_ w359]
                  tunnel: w318 -> [_ w360]
                  frame False {
                  }
                  frame True {
                    n146 = call "New-ExitCoords.vi"("LUT in"=w367, "correction trial"=w359, "Trials"=w360, "Blue/Yellow"=w366, "exit rad"=w374, "hab rad"=w375, "centroid"=w376, "center"=w377) -> ("LUT out"=w365:dbl[][], "output cluster 2"=w364:T33, "CW/CCW"=→"CW/CCW":bool, "output cluster"=w373:T38)
                    n147 = Tick Count (ms)() -> (millisecond timer value=w370:u32)
                    n148 = Replace Array Subset(array=w369, new element=w370, index=1) -> (w368:i32[])
                    n149 = Build Array (concatenate)(w362, w364) -> (w363:T35)
                  }
                }
                n150 = Select(t=69.0, s=w324, f=0.0) -> (s? t:f=w315:dbl)
                n151 = Replace Array Subset(array=dbl[] [0.0, 0.0, 0.0, 0.0], new element=w315, index=3) -> (w314:dbl[])
              }
              frame True {
                n152 = call "New-LUTindx.vi"("centroid"=w399, "exit angles"=w400, "center"=w398, "rad"=w397, "LUT"=w386) -> ("output"=w388:dbl[])  [unwired: 6 in]
                n153 = Compound Arithmetic op=OR(w382, w380, w392) -> (w395:bool)
                n154 = Or(x=w383, y=w393) -> (x .or. y?=w394:bool)
                n155 = Or(x=w395, y=w394) -> (x .or. y?=w396:bool)
                n156 = case shown="True" w396 {
                  selector: w396 -> [w402 _]
                  tunnel: w394 -> [_ w417]
                  tunnel: [TRUE FALSE] -> w391
                  tunnel: w385 -> [w405 w415]
                  tunnel: [w405 w414] -> w381
                  tunnel: w390 -> [w404 w413]
                  tunnel: [w404 w410] -> w389
                  tunnel: w380 -> [_ w409]
                  tunnel: [-1 w408] -> w379
                  tunnel: [w402 w407] -> w378
                  frame False {
                  }
                  frame True {
                    n157 = Tick Count (ms)() -> (millisecond timer value=w411:u32)
                    n158 = case shown="True" w417 {
                      selector: w417 -> [w418 _]
                      tunnel: w415 -> [w422 w442]
                      tunnel: [w421 w441] -> w414
                      tunnel: w409 -> [w420 _]
                      tunnel: [w419 0] -> w408
                      tunnel: [w418 w437] -> w407
                      frame False {
                        n159 = case shown="False" w420 {
                          tunnel: w422 -> [w429 w435]
                          tunnel: [w425 w431] -> w421
                          tunnel: [1 2] -> w419
                          frame False {
                            # "fail"
                            n160 = Index Array(array=w429) -> (element #1=w428:i32, element #2=w427:i32, element #3=w424:i32)  [unwired: 3 in]
                            n161 = Increment(x=w427) -> (x+1=w426:i32)
                            n162 = Replace Array Subset(array=w429, new element #1=w428, new element #2=w426, new element #3=w424) -> (w425:i32[])  [unwired: 3 in]
                          }
                          frame True {
                            # "omission"
                            n163 = Index Array(array=w435) -> (element #1=w436:i32, element #2=w434:i32, element #3=w433:i32)  [unwired: 3 in]
                            n164 = Increment(x=w433) -> (x+1=w432:i32)
                            n165 = Replace Array Subset(array=w435, new element #1=w436, new element #2=w434, new element #3=w432) -> (w431:i32[])  [unwired: 3 in]
                          }
                        }
                      }
                      frame True {
                        w438 = 0 ("new element/subarray")
                        # "success"
                        n166 = Index Array(array=w442) -> (element #1=w444:i32, element #2=w439:i32)  [unwired: 2 in]
                        n167 = Increment(x=w444) -> (x+1=w443:i32)
                        n168 = Greater?(x=w439, y=w438) -> (0:w437:bool)
                        n169 = Replace Array Subset(array=w442, new element #1=w443, new element #2=w438, new element #3=w438) -> (w441:i32[])  [unwired: 3 in]
                      }
                    }
                    n170 = Replace Array Subset(array=w413, new element=w411, index=1) -> (w410:i32[])
                  }
                }
              }
            }
            n171 = case "stop" shown="True" w275 {
              tunnel: w274 -> [_ w301]
              tunnel: w273 -> [_ w300]
              tunnel: [TRUE FALSE] -> w272
              tunnel: w207 -> [_ w297]
              tunnel: w206 -> [_ w296]
              tunnel: w197 -> [w293 _]
              tunnel: [w293 -1] -> w196
              frame False {
              }
              frame True {
                n172 = case shown="True" w301 {
                  tunnel: w300 -> [_ w303]
                  frame False {
                  }
                  frame True {
                    n173 = call "IMAQ AVI2 Close"("AVI Refnum"=w303) -> ()  [unwired: 10 in, 1 out]
                  }
                }
                n174 = case shown="True" w297 {
                  tunnel: w296 -> [_ w302]
                  frame False {
                  }
                  frame True {
                    n175 = call "IMAQ AVI2 Close"("AVI Refnum"=w302) -> ()  [unwired: 10 in, 1 out]
                  }
                }
                n176 = property on="Stop" class="Bool"("DisabledEnum"=T14."Disabled and Grayed Out" ("Disabled")) -> ()  [unwired: 2 in, 2 out]
              }
            }
            n177 = feedback-in #5(w196) -> ()
            n178 = Build Array (concatenate)(w260, w256, w259, w224, w255, w254, w204) -> (w237:dbl[])
            n179 = Build Array (concatenate)(w257, w237) -> (w242:dbl[][])
          }
        }
        "stimulus" <- w113
        "Trial #" <- w112
        "motor fb" <- w107
        "output" <- w73
        n180 = feedback-in #6("habituation") -> ()
        n181 = feedback #6("habituation") -> (w76:bool)
        n182 = Not Equal?(x="habituation", y=w76) -> (x != y?=w75:bool)
        n183 = case shown="True" w75 {
          tunnel: "habituation" -> [_ w165]
          frame False {
          }
          frame True {
            n184 = Select(t=T14."Disabled and Grayed Out" ("Disabled"), s=w165, f=T14."Enabled" ("Disabled")) -> (s? t:f=w162:T14)
            n185 = property on="trial settings" class="Clust (strict)"("DisabledEnum"=w162) -> ()  [unwired: 2 in, 2 out]
          }
        }
        n186 = case "save data" shown="True" w133 {
          tunnel: w90 -> [_ w609]
          tunnel: w97 -> [_ w605]
          tunnel: "dir" -> [_ w616]
          tunnel: w89 -> [_ w604]
          tunnel: w86 -> [_ w599]
          tunnel: "Controls" -> [_ w595]
          tunnel: "vid bandpass" -> [_ w566]
          tunnel: "exits" -> [_ w565]
          tunnel: "trial settings" -> [_ w569]
          tunnel: "feedback" -> [_ w570]
          tunnel: "habituation" -> [_ w540]
          frame False {
          }
          frame True {
            w574 = LVH5D_Operation."create or replace with confirmation" ("operation (open or create)")
            n187 = for {
              tunnel: w609 -> [w1154] mode=indexing
              tunnel: [w1153] -> w608 mode=indexing
              n188 = Index Array(array=w1154) -> (element #1=w1151:dbl, element #2=w1150:dbl, element #3=w1149:dbl, element #4=w1148:dbl, element #5=w1147:dbl, element #6=w1146:dbl, element #7=w1145:dbl, element #8=w1144:dbl, element #9=w1143:dbl, element #10=w1142:dbl, element #11=w1141:dbl, element #12=w1140:dbl, element #13=w1139:dbl, element #14=w1138:dbl, element #15=w1137:dbl)  [unwired: 15 in]
              n189 = Bundle(cluster=T22 {"Session Timer"=0.0, "Trial Timer"=0.0, "Trial #"=0.0, "Correction #"=0.0, "Omission"=0.0, "CentroidX"=0.0, "CentroidY"=0.0, "%Correct"=0.0, "%Incorrect"=0.0, "R"=0.0, "G"=0.0, "B"=0.0, "W"=0.0, "M"=0.0, "Total"=0.0}, "Session Timer"=w1151, "Trial Timer"=w1150, "Trial #"=w1149, "Correction #"=w1148, "Omission"=w1147, "CentroidX"=w1146, "CentroidY"=w1145, "%Correct"=w1144, "%Incorrect"=w1143, "R"=w1142, "G"=w1141, "B"=w1140, "W"=w1139, "M"=w1138, "Total"=w1137) -> (w1153:T22)
            }
            n190 = Unbundle(w565) -> ("hab scale"=w558:dbl, "exit radius (cm)"=w548:dbl, "% required in exit"=w547:dbl)
            n191 = Unbundle(w566) -> ("low1"=w564:i32, "high1"=w562:i32, "low2"=w561:i32, "high2"=w560:i32)
            n192 = Unbundle(w604) -> ("px2cm"=w572:dbl, "center"=w603:dbl[], "rad"=w545:dbl)  [unwired: 2 out]
            n193 = Unbundle(w616) -> ("Data Output Directory"=w615:path, "Session Name"=w614:string)
            n194 = Unbundle(w569) -> ("Num Trials"=w544:i32, "Trial Duration (s)"=w543:i32, "ITI (s)"=w542:i32, "incorrect ITI (s)"=w541:i32, "Total Timeout (s)"=w536:i32)
            n195 = Unbundle(w570) -> ("motor feedback mode"=w556:enum16{"constant", "time still"}, "min motor feedback"=w550:dbl, "max motor feedback"=w549:dbl, "max led feedback"=w554:dbl, "colormap"=w568:path)
            n196 = Index Array(array=w603) -> (element #1=w602:dbl, element #2=w601:dbl)  [unwired: 2 in]
            n197 = Concatenate Strings(w614, ".hdf5" ("string")) -> (w613:string)
            n198 = Format Into String(format string="trials=%d,duration=%d,ITI=%d,icITI=%d,timeout=%d", w544, w543, w542, w541, w536) -> (resulting string=w538:string)  [unwired: 2 in, 1 out]
            n199 = Format Into String(format string="L%dH%d,L%dH%d", w564, w562, w561, w560) -> (resulting string=w559:string)  [unwired: 2 in, 1 out]
            n200 = Format Into String(format string="mode=%s,min=%f,max=%f", w556, w550, w549) -> (resulting string=w555:string)  [unwired: 2 in, 1 out]
            n201 = Format Into String(format string="habScale=%f,exitRad=%f,required=%f", w558, w548, w547) -> (resulting string=w557:string)  [unwired: 2 in, 1 out]
            n202 = Build Path(base path=w615, name or relative path=w613) -> (appended path=w611:path)
            n203 = Unbundle By Name(w595) -> ("Rodent ID"=w594:i32, "Correct color"=w593:enum16{"UV", "Green"}, "poop count"=w592:i8)
            n204 = Format Into String(format string="X=%f,Y=%f,r=%f", w602, w601, w545) -> (resulting string=w590:string)  [unwired: 2 in, 1 out]
            n205 = Path To String(path=w568) -> (string=w567:string)
            n206 = Format Into String(w593) -> (resulting string=w596:string)  [unwired: 3 in, 1 out]
            n207 = Format Into String(w592) -> (resulting string=w591:string)  [unwired: 3 in, 1 out]
            n208 = Select(t="habituation", s=w540, f=w538) -> (s? t:f=w539:string)
            n209 = Format Into String(w554) -> (resulting string=w553:string)  [unwired: 3 in, 1 out]
            n210 = Format Into String(w594) -> (resulting string=w597:string)  [unwired: 3 in, 1 out]
            n211 = Format Into String(w572) -> (resulting string=w571:string)  [unwired: 3 in, 1 out]
            n212 = property on="attributes cluster" class="Clust (strict)"() -> ("Controls[]"=w607:refnum<vi>[])  [unwired: 2 in, 2 out]
            n213 = call <vilib>:"OpenCreateReplace HDF5 File.vi"("path"=w611) -> ("error out"=w580:errorcluster, "HDF5 Ref out"=w589:T39)  [unwired: 7 in]
            n214 = for {
              tunnel: w607 -> [w1136] mode=indexing
              tunnel: [w1135] -> w606 mode=indexing
              n215 = property class="Ctl"(reference=w1136) -> ("Label.Text"=w1135:string)  [unwired: 1 in, 2 out]
            }
            n216 = Bundle(cluster="attributes cluster", "timestamp"=w605, "ID"=w597, "correct color"=w596, "poop count"=w591, "trial settings"=w539, "motor settings"=w555, "max led fb"=w553, "colormap"=w567, "vid bandpass"=w559, "exit settings"=w557, "platform"=w590, "px2cm"=w571) -> (w573:T1)
            n217 = call-poly <vilib>:"OpenCreateGroup.vi"("Create if not found (F)"=TRUE, "error in (no error)"=w580, "Group"=w597, "HDF5 Ref"=w589) -> ("error out"=w579:errorcluster, "HDF5 Group Ref"=w586:T39, "HDF5 Ref out"=w581:T39)  [unwired: 5 in]
            n218 = xnode "Write Dataset with Attributes"("Dataset Path"="settings", "error in (no error)"=w579, "operation (open or create)"=w574, "HDF5 Path or Ref"=w586, "Attribute Name(s)"=w606, "Attribute Value(s)"=w573, "Data"=w599) -> ("HDF5 Ref out"=w585:T39, "error out"=w578:errorcluster)  [unwired: 1 in, 1 out]
            n219 = xnode "Simple H5Dwrite"("Dataset Path"="data", "error in (no error)"=w578, "operation (open or create)"=w574, "HDF5 Path or Ref"=w585, "Data"=w608) -> ("HDF5 Ref out"=w583:T39, "error out"=w577:errorcluster)  [unwired: 3 in, 1 out]
            n220 = call <vilib>:"H5Gclose.vi"("error in (no error)"=w577, "HDF5 Group Ref"=w583) -> ("error out"=w582:errorcluster)  [unwired: 7 in]
            n221 = call <vilib>:"H5Fclose.vi"("error in (no error)"=w582, "HDF5 Ref"=w581) -> ("error out"=w575:errorcluster)  [unwired: 7 in]
            n222 = call <vilib>:"Simple Error Handler.vi"("error source (\" \")"="save data path?" ("error source (\" \")"), "error in (no error)"=w575) -> ("error?"=w610:bool)  [unwired: 3 in, 4 out]
            n223 = case shown="False" w610 {
              tunnel: w594 -> [w1160 _]
              tunnel: w593 -> [w1159 _]
              frame False {
                w1155 = T14."Enabled" ("Disabled")
                n224 = Increment(x=w1159) -> (x+1=w1156:enum16{"UV", "Green"})
                n225 = Increment(x=w1160) -> (x+1=w1158:i32)
                n226 = property on="Start" class="Bool"("DisabledEnum"=w1155) -> ()  [unwired: 2 in, 2 out]
                n227 = property on="Stop" class="Bool"("DisabledEnum"=w1155) -> ()  [unwired: 2 in, 2 out]
                n228 = property on="Correct color" class="Enum (strict)"("Val(Sgnl)"=w1156) -> ()  [unwired: 2 in, 2 out]
                n229 = property on="poop count" class="DigNum (strict)"("Val(Sgnl)"=i8 0 ("Value (Signaling)")) -> ()  [unwired: 2 in, 2 out]
                n230 = property on="Rodent ID" class="DigNum (strict)"("Val(Sgnl)"=w1158) -> ()  [unwired: 2 in, 2 out]
              }
              frame True {
              }
            }
          }
        }
        n231 = case shown="False" w70 {
          tunnel: [w169 w183] -> w108
          tunnel: w73 -> [w176 _]
          tunnel: w58 -> [w175 w183]
          tunnel: w107 -> [w174 _]
          tunnel: w51 -> [w166 _]
          frame False {
            n232 = To Unsigned Byte Integer(number=w176) -> (unsigned 8bit integer=w172:u8[])
            n233 = call <vilib>:"Custom Command.vi"("Data"=w172, "Custom Command Number"=u16 0, "LINX Resource"=w175) -> ("LINX Resource"=w177:T27)  [unwired: 5 in, 3 out]
            n234 = call-poly <vilib>:"PWM Set Duty Cycle.vi"("Duty Cycle (0-1)"=w174, "PWM Channel"=u8 3, "LINX Resource"=w177) -> ("LINX Resource"=w170:T27)  [unwired: 7 in, 1 out]
            n235 = feedback-in #7(w166) -> ()
            n236 = feedback #7(FALSE) -> (w168:bool)
            n237 = case shown="True" w168 {
              tunnel: w170 -> [w178 w182]
              tunnel: [w178 w179] -> w169
              frame False {
              }
              frame True {
                n238 = call <vilib>:"Custom Command.vi"("Timeout (100 ms)"=1100, "Custom Command Number"=u16 1, "LINX Resource"=w182) -> ("LINX Resource"=w179:T27)  [unwired: 5 in, 3 out]
              }
            }
          }
          frame True {
          }
        }
        n239 = call "New-stim indicator.vi"("array"=w73) -> ("indicator"=w72:cluster{u32, u32}[])  [unwired: 10 in]
        n240 = property on="stimulus" class="Bool (strict)"("Colors [4]"=w72) -> ()  [unwired: 2 in, 2 out]
        n241 = disable-structure shown="Enabled" {
          frame Enabled {
            n242 = Tick Count (ms)() -> (millisecond timer value=w184:u32)
            n243 = feedback #8() -> (w185:u32)  [unwired: 1 in]
            n244 = Subtract(x=w184, y=w185) -> (x-y=→"x-y":u32)
            n245 = feedback-in #8(w184) -> ()
          }
          frame Disabled {
          }
        }
        n246 = node-c288() -> ()  [unwired: 1 in, 1 out]
      }
      n247 = node-c288(w49) -> ()  [unwired: 1 out]
      n248 = call <vilib>:"Close.vi"("LINX Resource"=w28) -> ()  [unwired: 10 in, 1 out]
      n249 = call "IMAQ Dispose"("Image"=w34) -> ()  [unwired: 5 in, 1 out]
      n250 = call "IMAQ Dispose"("Image"=w40) -> ()  [unwired: 5 in, 1 out]
      n251 = call <vilib>:"IMAQdx Close Camera.vi"("Session In"=w41) -> ()  [unwired: 10 in, 1 out]
    }
    frame #3 {
      n252 = case shown="True" "save settings to ini at close" {
        tunnel: w1170 -> [_ w1172]
        tunnel: w1169 -> [_ w1171]
        frame False {
        }
        frame True {
          n253 = for {
            tunnel: w1172 -> [w1174]
            tunnel: w1171 -> [w1173] mode=indexing
            n254 = call "my Write Controls on Tab to Config File.vi"("Page Refnum"=w1173, "configuration file path"=w1174) -> ()  [unwired: 4 in, 2 out]
          }
        }
      }
    }
  }
